vi "CuLab_Power_Spec_SGL.vi"(7 "window":u16(ring) items=["None "=0, "Hanning"=1, "Hamming"=2, "Blackman-Harris"=3, "Exact Blackman"=4, "Blackman"=5, "Flat Top"=6, "4 Term B-Harris "=7, "7 Term B-Harris"=8, "Low Sidelobe"=9, "Blackman Nuttall"=11], 8 "error in (no error)":errorcluster, 11 "T1D_SGL in":refnum<class "T1D_SGL.lvclass">) -> (0 "error out":errorcluster, 3 "Pwr Spec":refnum<class "T1D_SGL.lvclass">)   [LabVIEW 2020]
uses:
  <vilib>/Ngene/CuLab - GPU Accelerated Toolkit/Toolkit/Low_Level/Tensor_Classes/T_Children/T1D/T1D_Children/T1D_SGL/T1D_SGL.lvclass
  <vilib>/Ngene/CuLab - GPU Accelerated Toolkit/Toolkit/API/Signal Processing/Spectral/Power Spectrum/CU_Power_Spectrum_T1D_SGL.vi
  <vilib>/Ngene/CuLab - GPU Accelerated Toolkit/Toolkit/API/Numeric/Add/T1D/CU_AddC_T1D_SGL.vi
  <vilib>/Ngene/CuLab - GPU Accelerated Toolkit/Toolkit/API/Elementary/Exponential/Logarithm Base 10/T1D/CU_Logarithm_Base_10_T1D_SGL.vi
  <vilib>/Ngene/CuLab - GPU Accelerated Toolkit/Toolkit/API/Numeric/Multiply/T1D/CU_MultiplyC_T1D_SGL.vi
  <vilib>/Ngene/CuLab - GPU Accelerated Toolkit/Toolkit/CuLab.lvlib
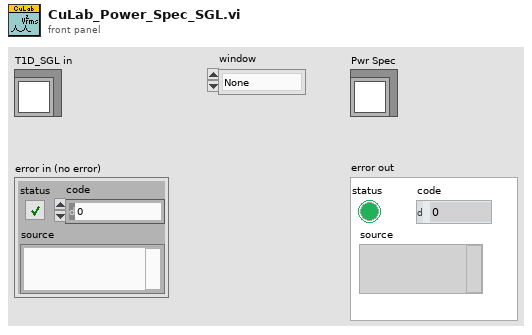
[diagram p1: front panel]
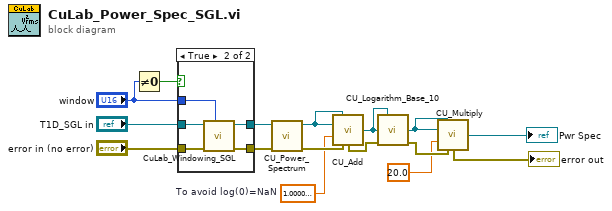
[diagram p0: block diagram]
diagram:
  w2 = sgl 1e-15  # To avoid log(0)=NaN
  n1 = Not Equal To 0?(x="window") -> (x != 0?=w10:bool)
  n2 = case shown="True" w10 {
    tunnel: "T1D_SGL in" -> [w18 w23]
    tunnel: [w18 w22] -> w7
    tunnel: "error in (no error)" -> [w17 w21]
    tunnel: [w17 w20] -> w6
    tunnel: "window" -> [_ w19]
    frame False {
    }
    frame True {
      n3 = call "CuLab_Windowing_SGL.vi"("window"=w19, "error in (no error)"=w21, "T1D_SGL in"=w23) -> ("error out"=w20:errorcluster, "T1D_SGL out"=w22:refnum<class "T1D_SGL.lvclass">)  [unwired: 7 in]
    }
  }
  n4 = call-poly <vilib>:"CU_Power_Spectrum.vi"("error in"=w6, "X"=w7) -> ("error out"=w5:errorcluster, "Power Spectrum"=w1:refnum<class "T1D_SGL.lvclass">)  [unwired: 8 in]
  n5 = call-poly <vilib>:"CU_Add.vi"("Dest in"=w1, "x"=w1, "y"=w2, "error in (no error)"=w5) -> ("Dest out"=w3:refnum<class "T1D_SGL.lvclass">, "error out"=w4:errorcluster)  [unwired: 10 in]
  n6 = call-poly <vilib>:"CU_Logarithm_Base_10.vi"("Dest in"=w3, "x"=w3, "error in (no error)"=w4) -> ("log(x)"=w14:refnum<class "T1D_SGL.lvclass">, "error out"=w16:errorcluster)  [unwired: 11 in]
  n7 = call-poly <vilib>:"CU_Multiply.vi"("Dest in"=w14, "x"=w14, "y"=sgl 20.0 ("f"), "error in (no error)"=w16) -> ("Dest out"=→"Pwr Spec":refnum<class "T1D_SGL.lvclass">, "error out"=→"error out":errorcluster)  [unwired: 10 in]
